vi "run.vi"(8 "error in (no error)":errorcluster, 11 "ImagingModeDL100901FlexTrajectory in":refnum<class "ImagingModeDL100901FlexTrajectory.lvclass">) -> (0 "error out":errorcluster, 3 "ImagingModeDL100901FlexTrajectory out":refnum<class "ImagingModeDL100901FlexTrajectory.lvclass">)   [LabVIEW 2010, in "ImagingModeDL100901FlexTrajectory.lvclass"]
uses:
  ImagingModeDL100901FlexTrajectory.lvclass
  main/labview_source/controls/undock_button.ctl
  common/xcontrols/XSettings/XSettings/XSettings.xctl
  common/classes/GenericComponent/GenericComponent/GenericComponent.lvclass
  ImagingModeDL100901FlexTrajectory.lvclass/ImagingModeDL100901FlexTrajectory.ctl
  ImagingModeDL091001Scaffold/ImagingModeDL091001Scaffold/ImagingModeDL091001Scaffold.lvclass
  ImagingModeDL091001Scaffold/ImagingModeDL091001Scaffold/internal_triggers_enum.ctl
  Trajectory/GenericTrajectory/GenericTrajectory/GenericTrajectory.lvclass
  common/classes/ErrorController/ErrorController/class_data.vi
  GenericImagingMode/GenericImagingMode/GenericImagingMode.lvclass
  common/classes/ErrorController/ErrorController/ErrorController.lvclass
panel:
  in  "button:undock?":T1
  in  "Tab Control":enum32{"User interface", "Debug", "About"}(tab)
  in  "XSettings":refnum<class "GenericComponent.lvclass">(xcontrol)
  in  "number of frames":i32
  out "frame counter":i32
  in  "defineTrajectoryButton":bool
  in  "pixel dwell time":dbl[unit]
  in  "scan rate":dbl[unit]=100.0
  in  "scan duration":dbl[unit]
  in  "scan repetitions":i32=1000
  in  "lines per frame":i32=200
  out "total number of \npixels per cycle":i32
  out "loaded settings?":bool
  out "finished?":bool
  out "event loop error":errorcluster
  out "event loop counter":i32
  out "ready for initialisation?":bool
  # "Scan parameters"
  # "Scan output"
  # "Visualization"
  # "ImagingModeDL100901FlexTrajectory\n\nImplemented by \n- Dominik Langer, University of Zurich, Switzerland\n- Chetan Nagaraja, Uppsala University, Sweden\n- Marcel van 't Hoff, University of Zurich, Switzerland"
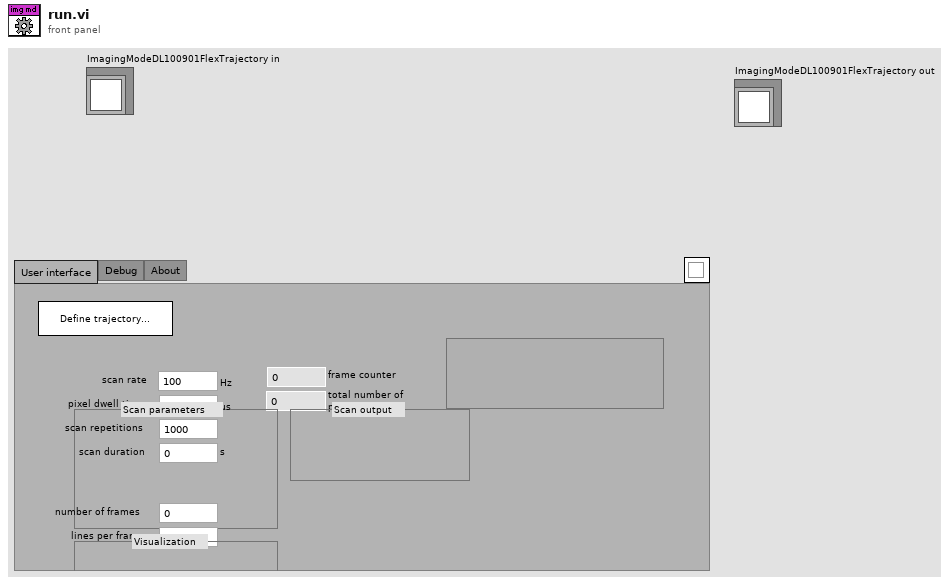
[diagram p1: front panel]
types:
  T1 = typedef "undock_button.ctl" = bool
  T2 = typedef "ImagingModeDL091001Scaffold.lvclass/internal_triggers_enum.ctl" = enum16{"NULL", "initialise", "terminate", "start sweep", "stop sweep", "update", "proceed", "draw overlay", "attach observer", "detach observer", "finish sweep"}
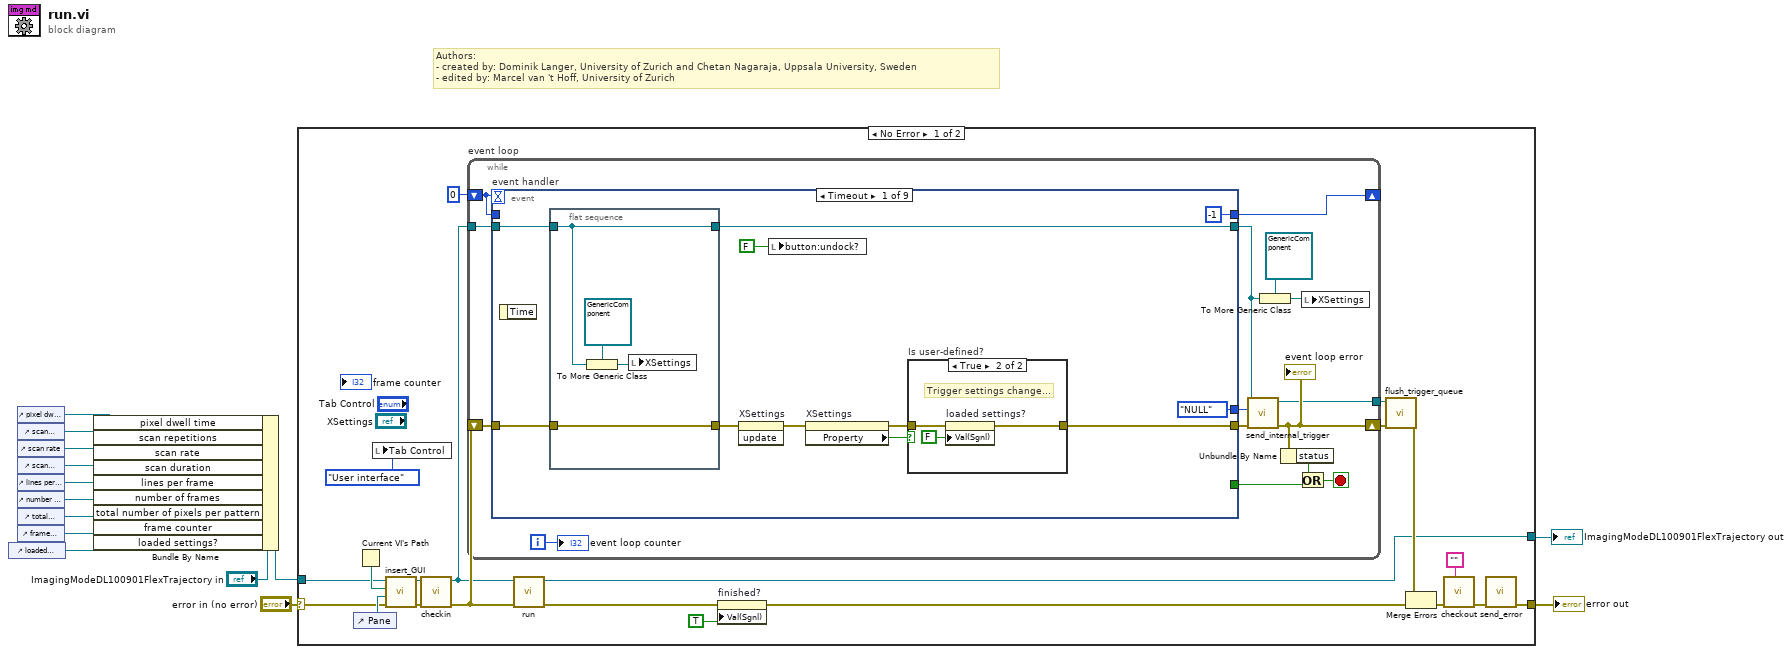
[diagram p0: block diagram]
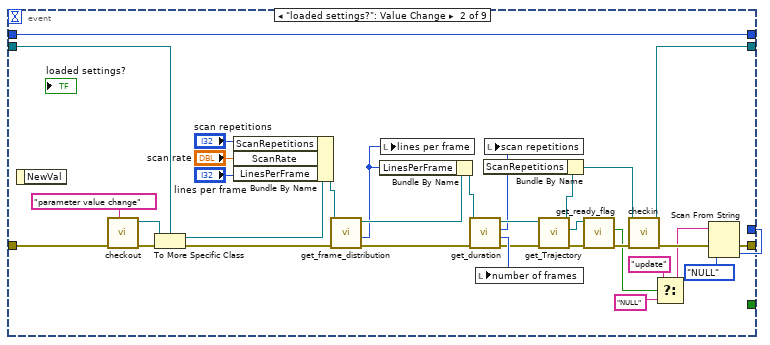
[diagram p3: hidden frame]
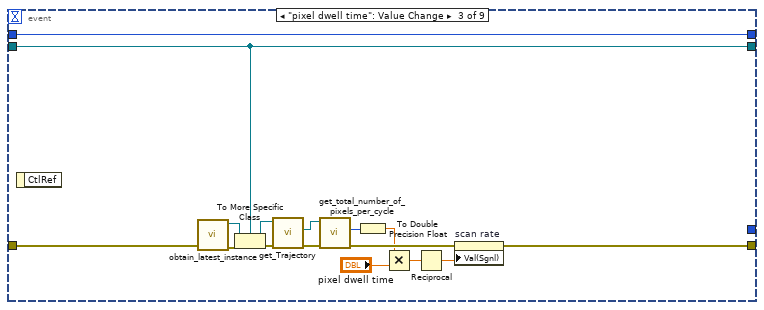
[diagram p4: hidden frame]
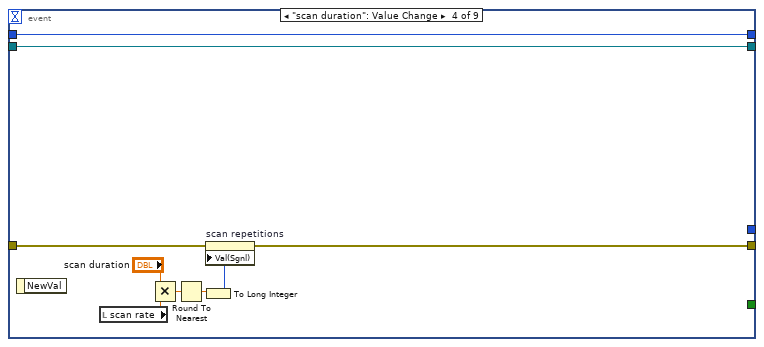
[diagram p5: hidden frame]
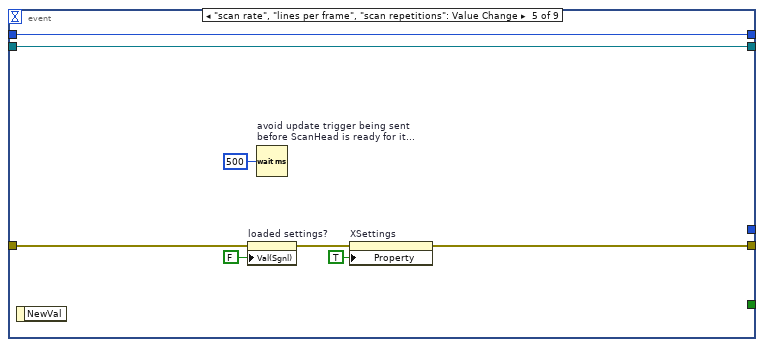
[diagram p6: hidden frame]
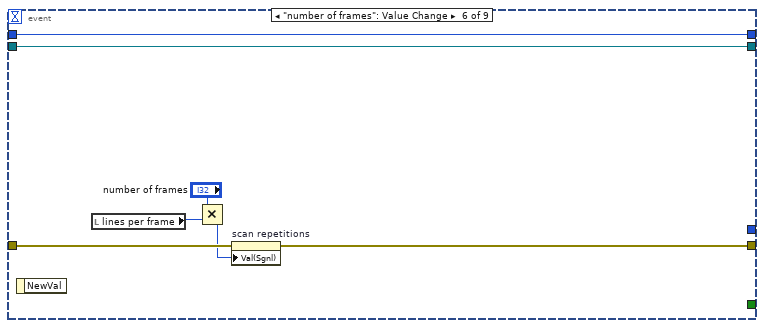
[diagram p7: hidden frame]
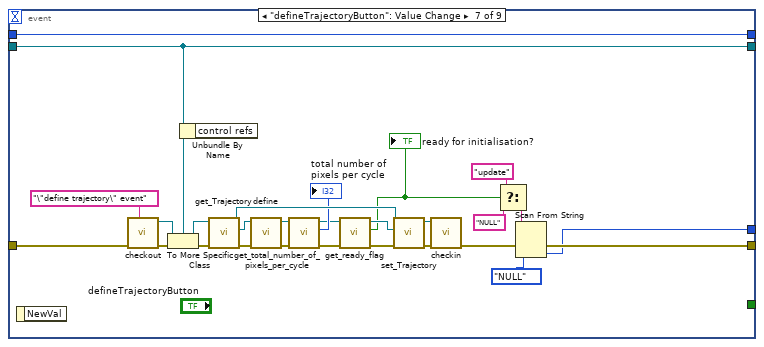
[diagram p8: hidden frame]
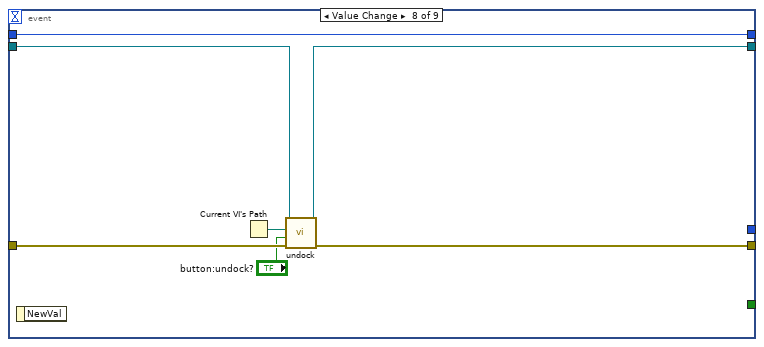
[diagram p9: hidden frame]
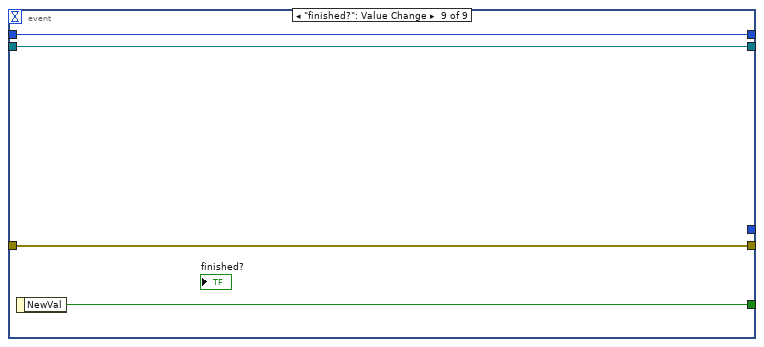
[diagram p10: hidden frame]
diagram:
  # "Authors: \n- created by: Dominik Langer, University of Zurich and Chetan Nagaraja, Uppsala University, Sweden\n- edited by: Marcel van 't Hoff, University of Zurich"
  n1 = control-ref of="loaded settings?"() -> (w1:refnum<vi>)
  n2 = control-ref of="pixel dwell time"() -> (w9:refnum<vi>)
  n3 = control-ref of="scan repetitions"() -> (w8:refnum<vi>)
  n4 = control-ref of="scan rate"() -> (w7:refnum<vi>)
  n5 = control-ref of="scan duration"() -> (w6:refnum<vi>)
  n6 = control-ref of="lines per frame"() -> (w5:refnum<vi>)
  n7 = control-ref of="number of frames"() -> (w2:refnum<vi>)
  n8 = control-ref of="total number of pixels per cycle"() -> (w3:refnum<vi>)
  n9 = control-ref of="frame counter"() -> (w4:refnum<vi>)
  n10 = Bundle By Name(cluster="ImagingModeDL100901FlexTrajectory in", "pixel dwell time"=w9, "scan repetitions"=w8, "scan rate"=w7, "scan duration"=w6, "lines per frame"=w5, "number of frames"=w2, "total number of pixels per pattern"=w3, "frame counter"=w4, "loaded settings?"=w1) -> (w11:refnum<class "ImagingModeDL100901FlexTrajectory.lvclass">)
  n11 = case shown="No Error" "error in (no error)" {
    selector: "error in (no error)" -> [w17 w184]
    tunnel: [w25 w184] -> w14
    tunnel: w11 -> [w18 w183]
    tunnel: [w15 w183] -> w12
    frame No Error {
      n12 = control-ref of="Pane"() -> (w29:refnum<vi>)
      n13 = Current VI's Path() -> (path=w31:path)
      n14 = local write "Tab Control"(enum32{"User interface", "Debug", "About"}."User interface" ("Tab Control")) -> ()
      n15 = call-dynamic "insert_GUI.vi"("error in (no error)"=w17, "Pane"=w29, "VI path"=w31, "GenericComponent in"=w18) -> ("error out"=w24:errorcluster, "GenericComponent out"=w16:refnum<class "ImagingModeDL100901FlexTrajectory.lvclass">)  [unwired: 6 in]
      n16 = call-dynamic "checkin.vi"("error in (no error)"=w24, "GenericScanMode in"=w16) -> ("error out"=w35:errorcluster, "GenericScanMode out"=w20:refnum<class "ImagingModeDL100901FlexTrajectory.lvclass">)  [unwired: 8 in]
      n17 = while "event loop" {
        shift-right: [w43] -> w22
        shift-left: w35 -> [w50]
        tunnel: w20 -> [w49]
        tunnel: [w42] -> w23
        shift-right: [w40] -> _
        shift-left: 0 -> [w41]
        i -> [w48]
        stop <- w44 stop-if-true
        n18 = event "event handler" shown="[0] Timeout" {
          selector: _ -> [_ _ _ _ _ _ _ _ _]
          dyn-events: _ -> [_ _ _ _ _ _ _ _ _]
          timeout: w41 -> [_ _ _ _ _ _ _ _ _]
          tunnel: w50 -> [w57 w76 w104 w126 w133 w141 w163 w175 w182]
          tunnel: [w51 w75 w106 w122 w130 w142 w146 w174 w182] -> w47
          tunnel: [_ _ _ _ _ _ _ _ w181] -> w46
          tunnel: [internal_triggers_enum."NULL" ("trigger") w74 _ _ _ _ w145 _ _] -> w39
          tunnel: w49 -> [w58 w73 w107 w121 w136 w138 w158 w177 w180]
          tunnel: [w56 w72 w107 w121 w136 w138 w158 w176 w180] -> w37
          tunnel: [-1 w103 w105 w120 w134 w137 w152 w178 w179] -> w40
          tunnel: w41 -> [_ w103 w105 w120 w134 w137 w152 w178 w179]
          event Timeout {
            n19 = event-data() -> ()  [unwired: 1 in, 1 out]
            n20 = flat-sequence {
              tunnel: w58 -> [w66]
              tunnel: w57 -> [w67]
              tunnel: [w67] -> w55
              tunnel: [w66] -> w56
              frame #0 {
                n21 = To More Generic Class(target class=refnum<class "GenericComponent.lvclass"> refnum ("GenericComponent.lvclass"), reference=w66) -> (generic class reference=w68:refnum<class "GenericComponent.lvclass">)
                n22 = local write "XSettings"(w68) -> ()
              }
            }
            n23 = invoke on="XSettings" class="XSettings (strict)" method="update"(error in=w55) -> (error out=w54:errorcluster)  [unwired: 2 in, 2 out]
            n24 = local write "button:undock?"(T1 FALSE ("button:undock?")) -> ()
            n25 = property on="XSettings" class="XSettings (strict)"(error in=w54) -> (error out=w53:errorcluster, "Property"=w52:bool)  [unwired: 1 in, 1 out]
            n26 = case "Is user-defined?" shown="True" w52 {
              tunnel: w53 -> [w62 w65]
              tunnel: [w62 w63] -> w51
              frame False {
              }
              frame True {
                # "Trigger settings change..."
                n27 = property on="loaded settings?" class="Bool (strict)"(error in=w65, "Val(Sgnl)"=FALSE ("Value (Signaling)")) -> (error out=w63:errorcluster)  [unwired: 1 in, 1 out]
              }
            }
          }
          event "loaded settings?": Value Change {
            n28 = event-data() -> ()  [unwired: 1 in, 1 out]
            n29 = call "checkout.vi"("locked by?"="parameter value change", "error in (no error)"=w76) -> ("error out"=w101:errorcluster, "GenericScanMode out"=w100:refnum<class "GenericImagingMode.lvclass">)  [unwired: 8 in]
            n30 = To More Specific Class(target class=w73, reference=w100, error in=w101) -> (specific class reference=w98:refnum<class "ImagingModeDL100901FlexTrajectory.lvclass">, error out=w95:errorcluster)
            n31 = Bundle By Name(cluster=w98, "ScanRepetitions"="scan repetitions", "ScanRate"="scan rate", "LinesPerFrame"="lines per frame") -> (w78:refnum<class "ImagingModeDL100901FlexTrajectory.lvclass">)
            n32 = call-dynamic "get_frame_distribution.vi"("error in (no error)"=w95, "ImagingModeDL100901FlexTrajectory in"=w78) -> ("error out"=w93:errorcluster, "lines per frame"=w71:i32, "ImagingModeDL100901FlexTrajectory out"=w77:refnum<class "ImagingModeDL100901FlexTrajectory.lvclass">)  [unwired: 6 in, 1 out]
            n33 = Bundle By Name(cluster=w77, "LinesPerFrame"=w71) -> (w94:refnum<class "ImagingModeDL100901FlexTrajectory.lvclass">)
            n34 = local write "lines per frame"(w71) -> ()
            n35 = call-dynamic "get_duration.vi"("error in (no error)"=w93, "ImagingModeDL100901FlexTrajectory in"=w94) -> ("error out"=w89:errorcluster, "number of frames"=w91:i32, "scan repetitions"=w70:i32, "ImagingModeDL100901FlexTrajectory out"=w86:refnum<class "ImagingModeDL100901FlexTrajectory.lvclass">)  [unwired: 6 in]
            n36 = local write "number of frames"(w91) -> ()
            n37 = local write "scan repetitions"(w70) -> ()
            n38 = call-dynamic "get_Trajectory.vi"("error in (no error)"=w89, "ScanModeDL090923Scaffold in"=w86) -> ("error out"=w88:errorcluster, "Trajectory"=w87:refnum<class "GenericTrajectory.lvclass">, "ScanModeDL090923Scaffold out"=w85:refnum<class "ImagingModeDL100901FlexTrajectory.lvclass">)  [unwired: 2 in, 5 out]
            n39 = Bundle By Name(cluster=w85, "ScanRepetitions"=w70) -> (w92:refnum<class "ImagingModeDL100901FlexTrajectory.lvclass">)
            n40 = call-dynamic "get_ready_flag.vi"("error in (no error)"=w88, "GenericTrajectory in"=w87) -> ("error out"=w90:errorcluster, "ready for initialisation?"=w84:bool)  [unwired: 7 in, 1 out]
            n41 = call-dynamic "checkin.vi"("error in (no error)"=w90, "GenericScanMode in"=w92) -> ("error out"=w83:errorcluster, "GenericScanMode out"=w72:refnum<class "ImagingModeDL100901FlexTrajectory.lvclass">)  [unwired: 8 in]
            n42 = Select(t="update", s=w84, f="NULL") -> (s? t:f=w80:string)
            n43 = Scan From String(input string=w80, error in=w83, default 1=internal_triggers_enum."NULL" ("trigger")) -> (error out=w75:errorcluster, output 1=w74:T2)  [unwired: 2 in, 2 out]
          }
          event "pixel dwell time": Value Change {
            n44 = event-data() -> ()  [unwired: 1 in, 1 out]
            n45 = call "obtain_latest_instance.vi"("error in (no error)"=w104) -> ("error out"=w118:errorcluster, "GenericScanMode out"=w117:refnum<class "GenericImagingMode.lvclass">)  [unwired: 9 in]
            n46 = To More Specific Class(target class=w107, reference=w117, error in=w118) -> (specific class reference=w116:refnum<class "ImagingModeDL100901FlexTrajectory.lvclass">, error out=w119:errorcluster)
            n47 = call-dynamic "get_Trajectory.vi"("error in (no error)"=w119, "ScanModeDL090923Scaffold in"=w116) -> ("error out"=w115:errorcluster, "Trajectory"=w114:refnum<class "GenericTrajectory.lvclass">)  [unwired: 2 in, 6 out]
            n48 = call-dynamic "get_total_number_of_pixels_per_cycle.vi"("error in (no error)"=w115, "GenericTrajectory in"=w114) -> ("error out"=w113:errorcluster, "total number of pixels per cycle"=w112:i32)  [unwired: 7 in, 1 out]
            n49 = To Double Precision Float(number=w112) -> (double precision float=w109:dbl)
            n50 = Multiply(x=w109, y="pixel dwell time") -> (x*y=w111:dbl[unit])
            n51 = Reciprocal(x=w111) -> (1/x=w110:dbl[unit])
            n52 = property on="scan rate" class="DigNum (strict)"(error in=w113, "Val(Sgnl)"=w110) -> (error out=w106:errorcluster)  [unwired: 1 in, 1 out]
          }
          event "scan duration": Value Change {
            n53 = event-data() -> ()  [unwired: 1 in, 1 out]
            n54 = local read "scan rate"() -> (w127:dbl[unit])
            n55 = Multiply(x="scan duration", y=w127) -> (x*y=w125:dbl)
            n56 = Round To Nearest(number=w125) -> (nearest integer value=w124:dbl)
            n57 = To Long Integer(number=w124) -> (32bit integer=w123:i32)
            n58 = property on="scan repetitions" class="DigNum (strict)"(error in=w126, "Val(Sgnl)"=w123) -> (error out=w122:errorcluster)  [unwired: 1 in, 1 out]
          }
          event "scan rate", "lines per frame", "scan repetitions": Value Change {
            n59 = event-data() -> ()  [unwired: 1 in, 1 out]
            n60 = property on="loaded settings?" class="Bool (strict)"(error in=w133, "Val(Sgnl)"=FALSE ("Value (Signaling)")) -> (error out=w131:errorcluster)  [unwired: 1 in, 1 out]
            n61 = Wait (ms) "avoid update trigger being sent\nbefore ScanHead is ready for it..."(milliseconds to wait=u32 500) -> ()  [unwired: 1 out]
            n62 = property on="XSettings" class="XSettings (strict)"(error in=w131, "Property"=TRUE ("is user-defined?")) -> (error out=w130:errorcluster)  [unwired: 1 in, 1 out]
          }
          event "number of frames": Value Change {
            n63 = event-data() -> ()  [unwired: 1 in, 1 out]
            n64 = local read "lines per frame"() -> (w140:i32)
            n65 = Multiply(x="number of frames", y=w140) -> (x*y=w139:i32)
            n66 = property on="scan repetitions" class="DigNum (strict)"(error in=w141, "Val(Sgnl)"=w139) -> (error out=w142:errorcluster)  [unwired: 1 in, 1 out]
          }
          event "defineTrajectoryButton": Value Change {
            n67 = event-data() -> ()  [unwired: 1 in, 1 out]
            n68 = call "checkout.vi"("locked by?"="\"define trajectory\" event", "error in (no error)"=w163) -> ("error out"=w169:errorcluster, "GenericScanMode out"=w170:refnum<class "GenericImagingMode.lvclass">)  [unwired: 8 in]
            n69 = To More Specific Class(target class=w158, reference=w170, error in=w169) -> (specific class reference=w162:refnum<class "ImagingModeDL100901FlexTrajectory.lvclass">, error out=w168:errorcluster)
            n70 = Unbundle By Name(w158) -> ()  [unwired: 1 out]
            n71 = call-dynamic "get_Trajectory.vi"("error in (no error)"=w168, "ScanModeDL090923Scaffold in"=w162) -> ("error out"=w160:errorcluster, "Trajectory"=w161:refnum<class "GenericTrajectory.lvclass">, "ScanModeDL090923Scaffold out"=w167:refnum<class "ImagingModeDL100901FlexTrajectory.lvclass">)  [unwired: 2 in, 5 out]
            n72 = call-dynamic "define.vi"("error in (no error)"=w160, "GenericTrajectory in"=w161) -> ("error out"=w159:errorcluster, "GenericTrajectory out"=w157:refnum<class "GenericTrajectory.lvclass">)  [unwired: 8 in]
            n73 = call-dynamic "get_total_number_of_pixels_per_cycle.vi"("error in (no error)"=w159, "GenericTrajectory in"=w157) -> ("error out"=w155:errorcluster, "total number of pixels per cycle"=→"total number of \npixels per cycle":i32, "GenericTrajectory out"=w156:refnum<class "GenericTrajectory.lvclass">)  [unwired: 7 in]
            n74 = call-dynamic "get_ready_flag.vi"("error in (no error)"=w155, "GenericTrajectory in"=w156) -> ("error out"=w154:errorcluster, "ready for initialisation?"=w148:bool, "GenericTrajectory out"=w153:refnum<class "GenericTrajectory.lvclass">)  [unwired: 7 in]
            "ready for initialisation?" <- w148
            n75 = call-dynamic "set_Trajectory.vi"("error in (no error)"=w154, "GenericTrajectory.lvclass"=w153, "ScanModeDL090923Scaffold in"=w167) -> ("error out"=w171:errorcluster, "ScanModeDL090923Scaffold out"=w166:refnum<class "ImagingModeDL100901FlexTrajectory.lvclass">)  [unwired: 7 in]
            n76 = call-dynamic "checkin.vi"("error in (no error)"=w171, "GenericScanMode in"=w166) -> ("error out"=w147:errorcluster)  [unwired: 8 in, 1 out]
            n77 = Select(t="update", s=w148, f="NULL") -> (s? t:f=w144:string)
            n78 = Scan From String(input string=w144, error in=w147, default 1=internal_triggers_enum."NULL" ("trigger")) -> (error out=w146:errorcluster, output 1=w145:T2)  [unwired: 2 in, 2 out]
          }
          event Value Change {
            n79 = event-data() -> ()  [unwired: 1 in, 1 out]
            n80 = Current VI's Path() -> (path=w173:path)
            n81 = call-dynamic "undock.vi"("error in (no error)"=w175, "undock?"="button:undock?", "VI path"=w173, "component in"=w177) -> ("error out"=w174:errorcluster, "component out"=w176:refnum<class "ImagingModeDL100901FlexTrajectory.lvclass">)  [unwired: 6 in]
          }
          event "finished?": Value Change {
            n82 = event-data() -> ("NewVal"=w181:bool)  [unwired: 1 in]
          }
        }
        n83 = call-dynamic "send_internal_trigger.vi"("error in"=w47, "trigger"=w39, "ScanModeDL091001Scaffold in"=w37) -> ("error out"=w43:errorcluster, "ScanModeDL091001Scaffold out"=w42:refnum<class "ImagingModeDL100901FlexTrajectory.lvclass">)  [unwired: 7 in]
        "event loop error" <- w43
        n84 = To More Generic Class(target class=refnum<class "GenericComponent.lvclass"> refnum ("GenericComponent.lvclass"), reference=w37) -> (generic class reference=w36:refnum<class "GenericComponent.lvclass">)
        n85 = Unbundle By Name(w43) -> ("status"=w45:bool)
        n86 = Or(x=w45, y=w46) -> (x .or. y?=w44:bool)
        n87 = local write "XSettings"(w36) -> ()
        "event loop counter" <- w48
      }
      n88 = call-parent "run.vi"("error in (no error)"=w35, "ScanModeDL091001Scaffold in"=w20) -> ("error out"=w34:errorcluster, "ScanModeDL091001Scaffold out"=w15:refnum<class "ImagingModeDL100901FlexTrajectory.lvclass">)  [unwired: 8 out]
      n89 = property on="finished?" class="Bool (strict)"(error in=w34, "Val(Sgnl)"=TRUE) -> (error out=w28:errorcluster)  [unwired: 1 in, 1 out]
      n90 = call-dynamic "flush_trigger_queue.vi"("error in (no error)"=w22, "GenericToplevelComponent in"=w23) -> ("error out"=w21:errorcluster)  [unwired: 8 in, 1 out]
      n91 = Merge Errors(w21, w28) -> (w27:errorcluster)
      n92 = call "checkout.vi"("locked by?"="", "error in (no error)"=w27) -> ("error out"=w26:errorcluster)  [unwired: 8 in, 1 out]
      n93 = call "send_error.vi"("error in (no error)"=w26) -> ("error out"=w25:errorcluster)  [unwired: 10 in]
    }
    frame Error {
    }
  }
  "error out" <- w14
  "ImagingModeDL100901FlexTrajectory out" <- w12
